vi "Excel(F)_dev.vi"(0 "Master Path":path, 1 "Excel File Name :":string, 2 "Protected?":bool, 3 "Password":string, 11 "error in (no error)":errorcluster, 12 "Filter":bool, 13 "eData":T1(array[cluster])) -> (15 "error out":errorcluster)   [LabVIEW 2020]
uses:
  <vilib>/Utility/miscctls.llb/LVPointTypeDef.ctl
  <userlib>/_Correct File Name/_correct file name.vi
panel:
  in  "Hide":bool
  in  "Cancel":bool
  in  "Save":bool
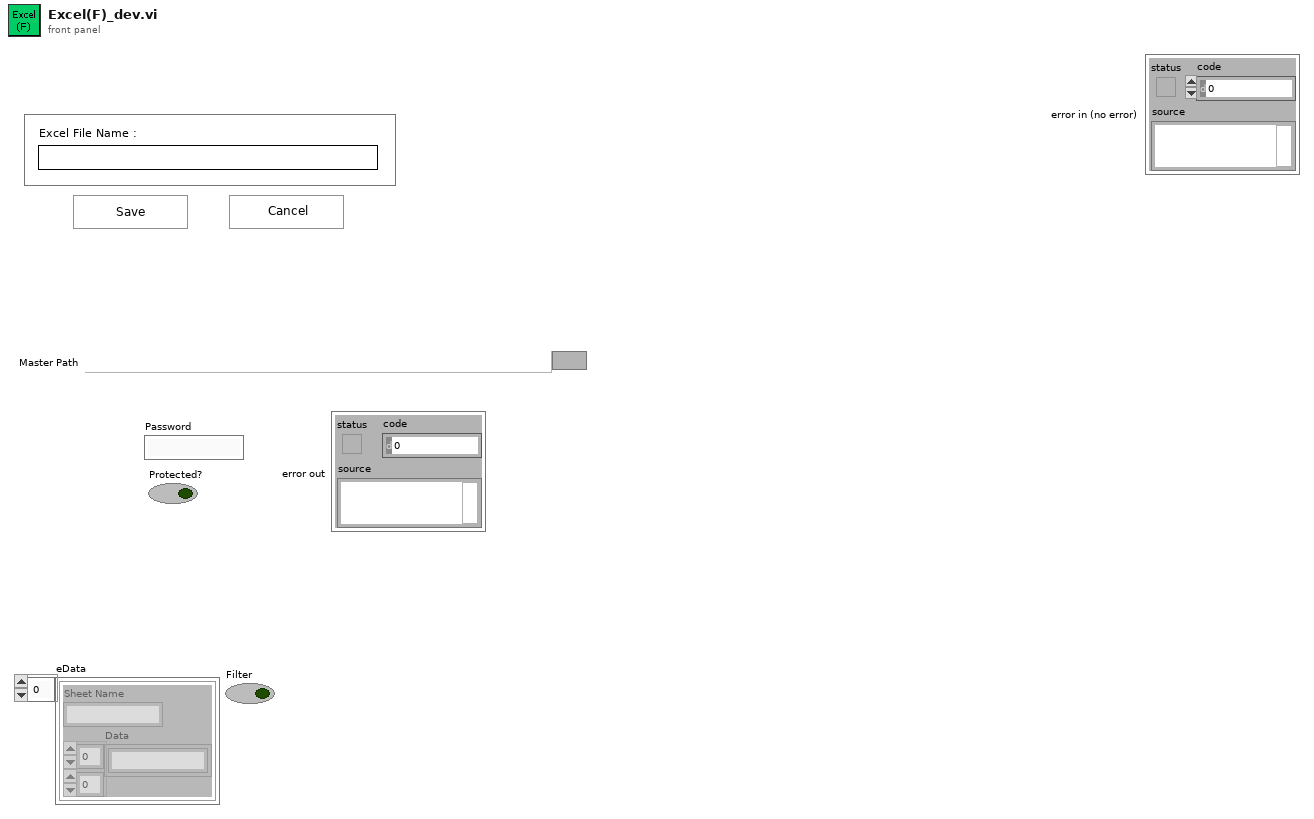
[diagram p1: front panel]
types:
  T1 = cluster{"Sheet Name":string, "Data":string[][]}[]
  T2 = typedef "LVPointTypeDef.ctl" = cluster{"Horizontal":i16, "Vertical":i16}
  T3 = cluster{"Data Path":path, "Calibration Path":path, "Settings Path":path, "Script Path":path, "DAQ Support":path, "Reporting Desktop":path, "Help":path}
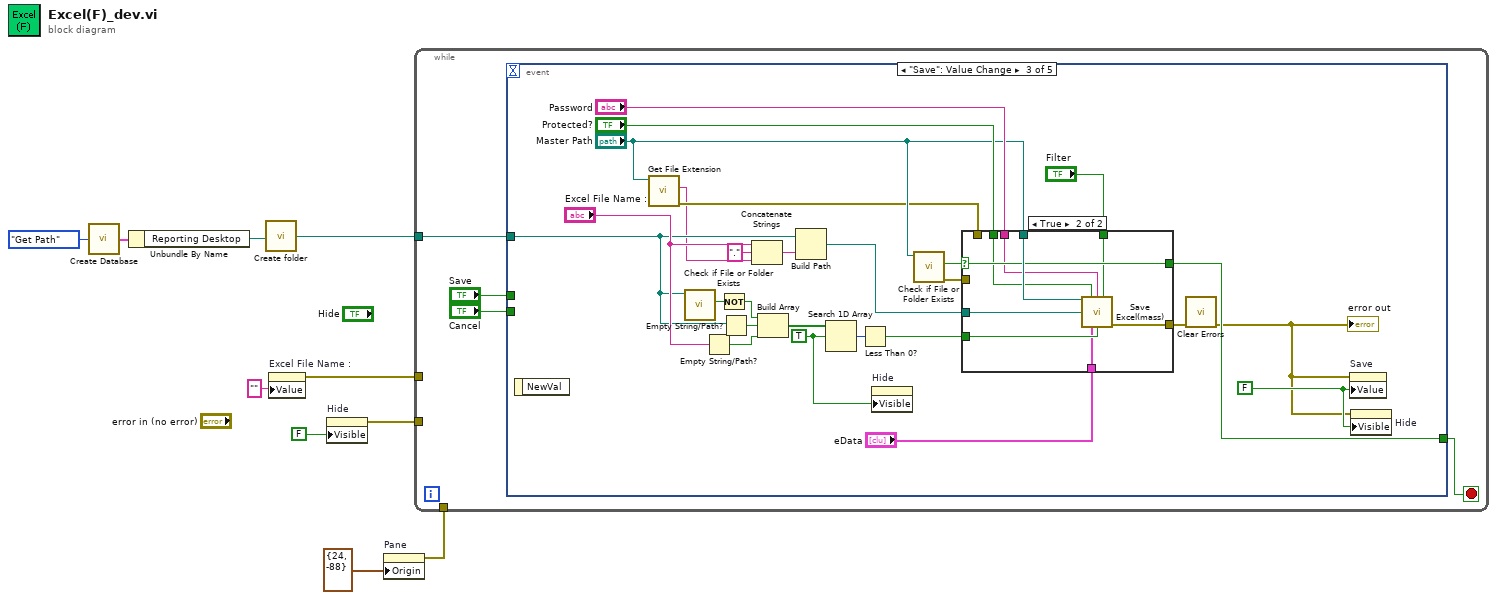
[diagram p0: block diagram]
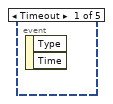
[diagram p2: hidden frame]
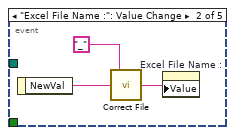
[diagram p3: hidden frame]
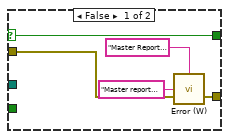
[diagram p4: hidden frame]
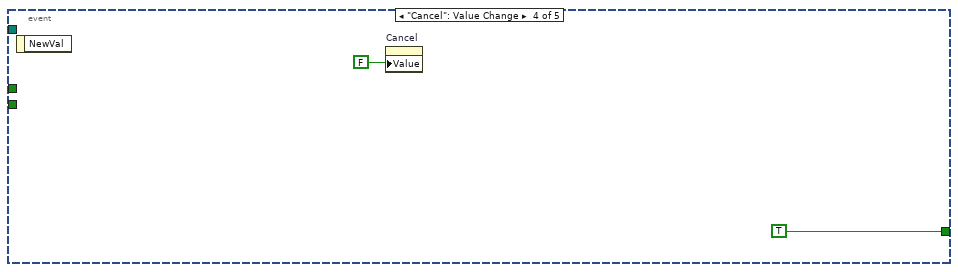
[diagram p5: hidden frame]
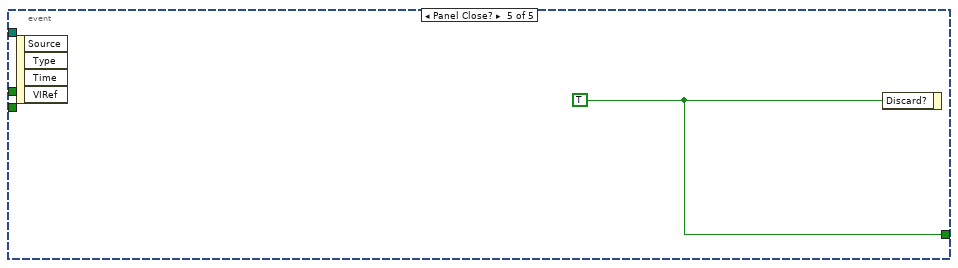
[diagram p6: hidden frame]
diagram:
  n1 = call <userlib>:"Create Database.vi"("Get/Create"=enum16{"Get Path", "Create Path"}."Get Path") -> ("Path Out"=w5:T3)  [unwired: 13 in, 1 out]
  n2 = Unbundle By Name(w5) -> ("Reporting Desktop"=w4:path)
  n3 = call <userlib>:"Create folder.vi"("Path In"=w4) -> ("Path out"=w3:path)  [unwired: 14 in]
  n4 = property on="Excel File Name :" class="Str"("Value"="" ("Excel File Name :")) -> (error out=w10:errorcluster)  [unwired: 2 in, 1 out]
  n5 = property on="Hide" class="Bool"("Visible"=FALSE ("Save")) -> (error out=w7:errorcluster)  [unwired: 2 in, 1 out]
  n6 = property on="Pane" class="Pane"("Origin"=T2 {"Horizontal"=24, "Vertical"=-88}) -> (error out=w1:errorcluster)  [unwired: 2 in, 1 out]
  n7 = while {
    tunnel: w10 -> [_]
    tunnel: w7 -> [_]
    tunnel: w3 -> [w11]
    tunnel: w1 -> [_]
    stop <- w12 stop-if-true
    n8 = event shown="[2] \"Save\": Value Change" {
      selector: _ -> [_ _ _ _ _]
      dyn-events: _ -> [_ _ _ _ _]
      timeout: _ -> [_ _ _ _ _]
      tunnel: "Save" -> [_ _ _ _ _]
      tunnel: "Cancel" -> [_ _ _ _ _]
      tunnel: [_ _ w28 TRUE ("Save") w59] -> w12
      tunnel: w11 -> [_ _ w26 _ _]
      event Timeout {
        n9 = event-data() -> ()  [unwired: 1 in, 2 out]
      }
      event "Excel File Name :": Value Change {
        n10 = event-data() -> ("NewVal"=w17:string)  [unwired: 1 in]
        n11 = call-poly <userlib>:"Correct File.vi"("Replace Char"="_", "File Name"=w17) -> ("File Name out"=w15:string)  [unwired: 13 in]
        n12 = property on="Excel File Name :" class="Str"("Value"=w15) -> ()  [unwired: 2 in, 2 out]
      }
      event "Save": Value Change {
        w31 = FALSE ("Save")
        w33 = TRUE ("element")
        n13 = event-data() -> ()  [unwired: 1 in, 1 out]
        n14 = call <vilib>:"Get File Extension.vi"("file"="Master Path") -> ("error out"=w22:errorcluster, "lowercase file extension"=w21:string)  [unwired: 6 in, 3 out]
        n15 = call <vilib>:"Check if File or Folder Exists.vi"("path"=w26) -> ("file or folder exists?"=w39:bool)  [unwired: 8 in, 2 out]
        n16 = Empty String/Path?(string/path="Excel File Name :") -> (empty?=w36:bool)
        n17 = Not(x=w39) -> (.not. x?=w38:bool)
        n18 = Empty String/Path?(string/path=w26) -> (empty?=w37:bool)
        n19 = Concatenate Strings("Excel File Name :", "." ("string"), w21) -> (w40:string)
        n20 = Build Array(w38, w37, w36) -> (w35:bool[])
        n21 = Build Path(base path=w26, name or relative path=w40) -> (appended path=w42:path)
        n22 = Search 1D Array(1D array=w35, element=w33) -> (index of element=w34:i32)  [unwired: 1 in]
        n23 = Less Than 0?(x=w34) -> (x < 0?=w43:bool)
        n24 = property on="Hide" class="Bool"("Visible"=w33) -> ()  [unwired: 2 in, 2 out]
        n25 = call <vilib>:"Check if File or Folder Exists.vi"("path"="Master Path") -> ("error out"=w29:errorcluster, "file or folder exists?"=w30:bool)  [unwired: 8 in, 1 out]
        n26 = case shown="True" w30 {
          selector: w30 -> [w47 w53]
          tunnel: w43 -> [_ w56]
          tunnel: w42 -> [_ w55]
          tunnel: [w46 w52] -> w32
          tunnel: "Master Path" -> [_ w54]
          tunnel: w29 -> [w46 _]
          tunnel: [w47 w53] -> w28
          tunnel: "Protected?" -> [_ w51]
          tunnel: "Password" -> [_ w50]
          tunnel: w22 -> [_ _]
          tunnel: "eData" -> [_ w49]
          tunnel: "Filter" -> [_ w48]
          frame False {
            n27 = call <userlib>:"Error (W).vi"("Title"="Master Report Error !!!", "Warning in"="Master report excel file is missing, check that & try again.") -> ()  [unwired: 14 in]
          }
          frame True {
            n28 = call "Save Excel(mass).vi"("Master Report Path"=w54, "Protected?"=w51, "Password"=w50, "Filter"=w48, "Save Path"=w55, "eData"=w49, "OK"=w56) -> ("error out"=w52:errorcluster)  [unwired: 7 in, 1 out]
          }
        }
        n29 = call <vilib>:"Clear Errors.vi"("error in (no error)"=w32) -> ("error out"=w27:errorcluster)  [unwired: 5 in, 1 out]
        "error out" <- w27
        n30 = property on="Save" class="Bool (strict)"(error in=w27, "Value"=w31) -> ()  [unwired: 1 in, 2 out]
        n31 = property on="Hide" class="Bool"(error in=w27, "Visible"=w31) -> ()  [unwired: 1 in, 2 out]
      }
      event "Cancel": Value Change {
        n32 = event-data() -> ()  [unwired: 1 in, 1 out]
        n33 = property on="Cancel" class="Bool (strict)"("Value"=FALSE ("Cancel")) -> ()  [unwired: 2 in, 2 out]
      }
      event Panel Close? {
        w59 = TRUE ("Discard?")
        n34 = event-data() -> ()  [unwired: 1 in, 4 out]
        n35 = event-data("Discard?"=w59) -> ()  [unwired: 1 in, 1 out]
      }
    }
  }
